vi "Wire Handle Messages Case.vi"(8 "error in (no error)":errorcluster, 11 "Setter Generator In":refnum<class "Setter Generator.lvclass">) -> (0 "error out":errorcluster, 3 "Setter Generator Out":refnum<class "Setter Generator.lvclass">)   [LabVIEW 2020, in "Method Generation.lvlib" / "Setter Generator.lvclass"]
uses:
  Setter Generator.lvclass
  Setter Generator.lvclass/Setter Generator.ctl
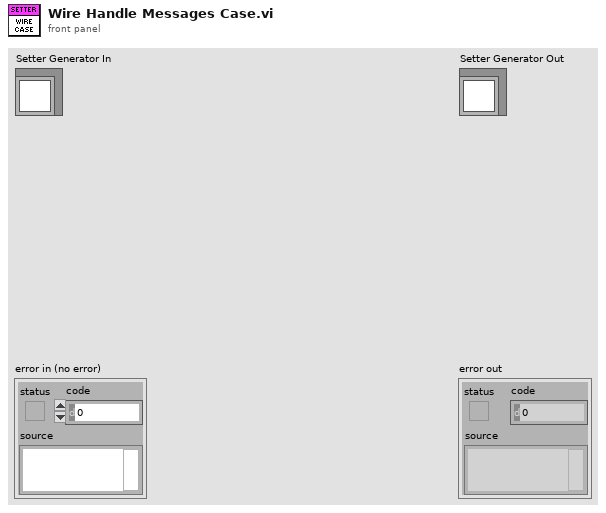
[diagram p1: front panel]
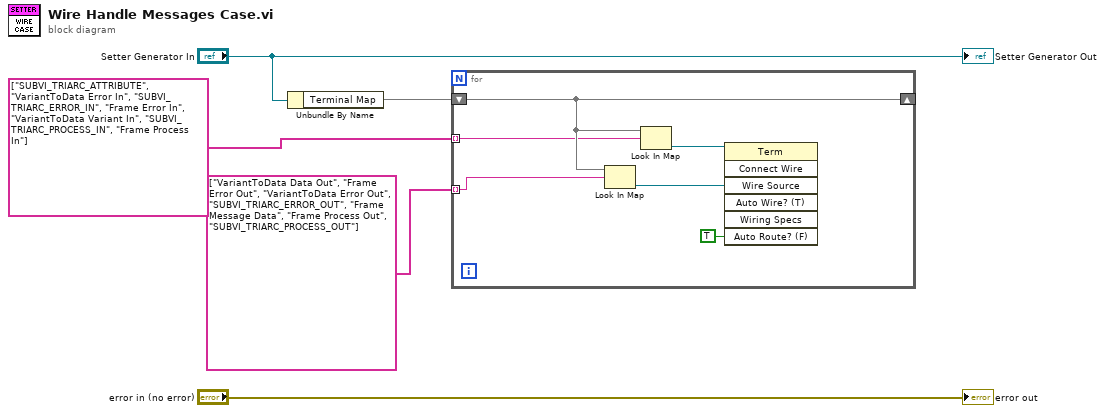
[diagram p0: block diagram]
diagram:
  n1 = Unbundle By Name("Setter Generator In") -> ("Terminal Map"=w3:map{string, refnum<vi>})
  n2 = for {
    shift-right: [w11] -> _
    shift-left: w3 -> [w11]
    tunnel: string[] ["SUBVI_TRIARC_ATTRIBUTE", "VariantToData Error In", "SUBVI_TRIARC_ERROR_IN", "Frame Error In", "VariantToData Variant In", "SUBVI_TRIARC_PROCESS_IN", "Frame Process In"] ("key") -> [w10] mode=indexing
    tunnel: string[] ["VariantToData Data Out", "Frame Error Out", "VariantToData Error Out", "SUBVI_TRIARC_ERROR_OUT", "Frame Message Data", "Frame Process Out", "SUBVI_TRIARC_PROCESS_OUT"] ("key") -> [w9] mode=indexing
    n3 = Look In Map(map=w11, key=w9) -> (value=w7:refnum<vi>)  [unwired: 1 in, 1 out]
    n4 = Look In Map(map=w11, key=w10) -> (value=w8:refnum<vi>)  [unwired: 1 in, 1 out]
    n5 = invoke class="Term" method="Connect Wire"(reference=w8, "Wire Source"=w7, "Auto Route? (F)"=TRUE) -> ()  [unwired: 4 in, 7 out]
  }
  "error out" <- "error in (no error)"
  "Setter Generator Out" <- "Setter Generator In"
